vi "Group Count.vi"(8 "error in (no error)":errorcluster, 11 "Thread Configuration in":refnum<class "Thread Configuration.lvclass">) -> (0 "error out":errorcluster, 2 "group count":i32, 3 "Thread Configuration out":refnum<class "Thread Configuration.lvclass">)   [LabVIEW 2019, in "DSF Core.lvlib" / "Thread Configuration.lvclass"]
uses:
  Thread Configuration.lvclass
  Thread Configuration.lvclass/Thread Configuration.ctl
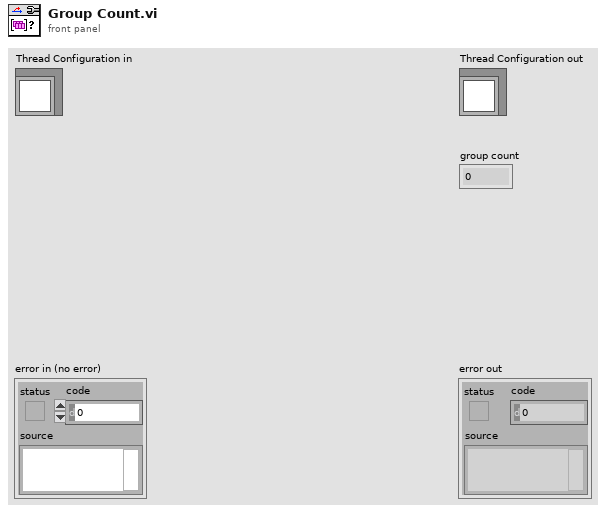
[diagram p1: front panel]
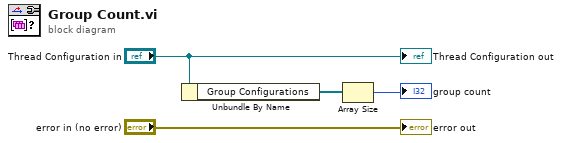
[diagram p0: block diagram]
diagram:
  n1 = Unbundle By Name("Thread Configuration in") -> ("Group Configurations"=w3:refnum<class "Group Configuration.lvclass">[])
  n2 = Array Size(array=w3) -> (size(s)=→"group count":i32)
  "error out" <- "error in (no error)"
  "Thread Configuration out" <- "Thread Configuration in"
